vi "_RT Read XML Expt.vi"(4 "error in":errorcluster, 6 "# of Expts":i32, 7 "XML String":string) -> (0 "error out":errorcluster, 1 "Expt":T1[](array[typedef]) {"ScanType" format="%#.6g"; "Mass Range"."Res" items=["High/High", "Medium/Medium", "Low/Low", "High/Medium", "High/Low", "Medium/High", "Medium/Low", "Low/High", "Low/Medium"]}, 3 "Remaining String":string)   [LabVIEW 2015]
uses:
  Type/_XML Expt.ctl
  Type/_XML Lens.ctl
  Type/_Mass Range Property.ctl
  Type/_Mass Range Parameters.ctl
  Type/_RT Res Type.ctl
  Type/_XML Type.ctl
  _RT Global.vi
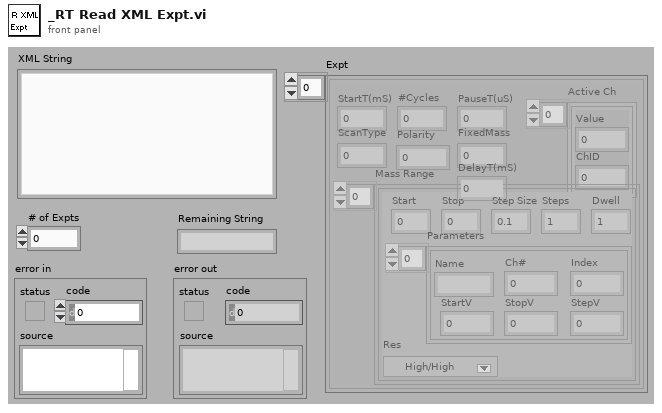
[diagram p1: front panel]
types:
  T1 = typedef "_XML Expt.ctl" = cluster{"StartT(mS)":i32, "#Cycles":i32, "PauseT(uS)":i32, "ScanType":i32, "Polarity":u8, "FixedMass":dbl, "DelayT(mS)":i32, "Active Ch":T2[], "Mass Range":T3[]}
  T2 = typedef "_XML Lens.ctl" = cluster{"Value":dbl, "ChID":u8}
  T3 = typedef "_Mass Range Property.ctl" = cluster{"Start":dbl, "Stop":dbl, "Step Size":dbl, "Steps":i32, "Dwell":dbl, "Parameters":T4[], "Res":T5}
  T4 = typedef "_Mass Range Parameters.ctl" = cluster{"Name":string, "Ch#":u8, "StartV":dbl, "StopV":dbl, "StepV":dbl, "Index":u8}
  T5 = typedef "_RT Res Type.ctl" = u16
  T6 = typedef "_XML Type.ctl" = enum16{"Configuration", "ConTable", "Method", "Experiment", "Mass Range", "Table", "LensTable", "ParamTable", "TuneParam", "MetParam", "MassRange", "LCMethod", "LCMethodFile", "RackType", "Vial", "PlatePos", "InjVol"}
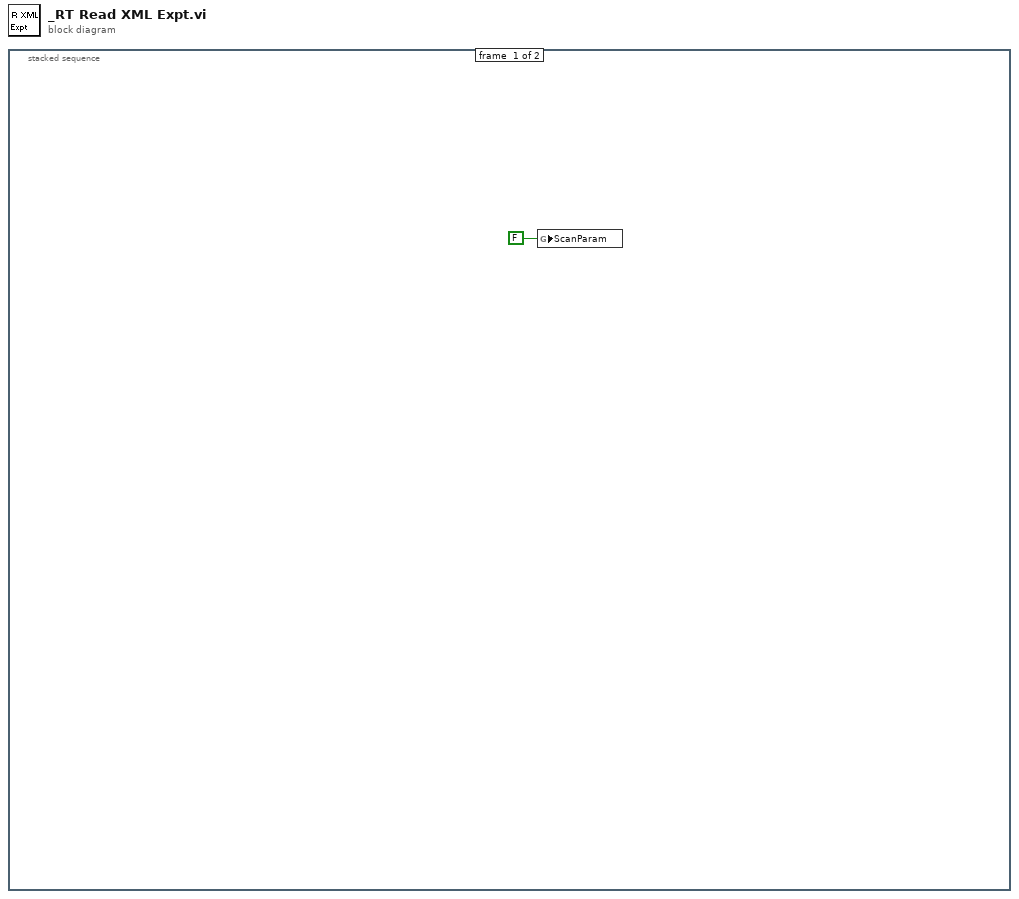
[diagram p0: block diagram]
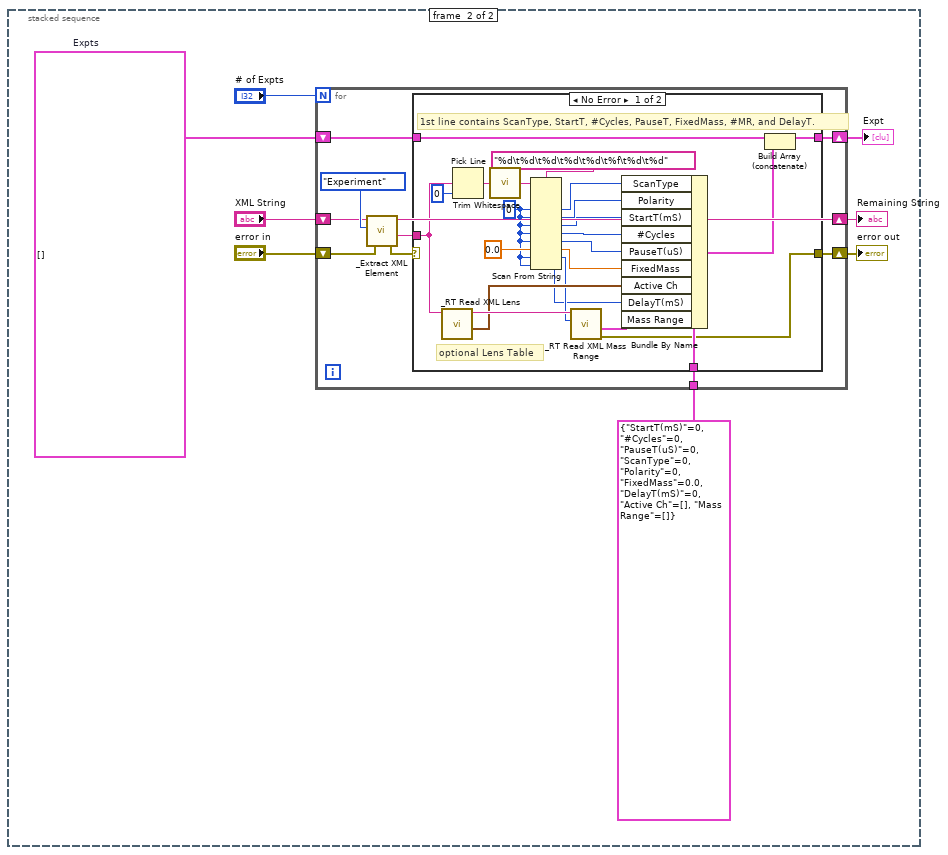
[diagram p2: hidden frame]
diagram:
  n1 = stacked-sequence {
    frame #0 {
      n2 = global write "_RT Global.vi" "ScanParam"(FALSE ("ScanParam")) -> ()
    }
    frame #1 {
      w4 = T1[] []  # Expts
      n3 = for {
        N: "# of Expts" -> [_]
        shift-right: [w13] -> w6
        shift-left: "XML String" -> [w15]
        shift-right: [w14] -> w5
        shift-left: "error in" -> [w18]
        shift-right: [w10] -> w2
        shift-left: w4 -> [w12]
        tunnel: T1 {"StartT(mS)"=0, "#Cycles"=0, "PauseT(uS)"=0, "ScanType"=0, "Polarity"=0, "FixedMass"=0.0, "DelayT(mS)"=0, "Active Ch"=[], "Mass Range"=[]} ("Expt") -> [w11]
        n4 = call "_Extract XML Element.vi"("error in"=w18, "XML Type"=_XML_Type."Experiment", "XML String"=w15) -> ("error out"=w17:errorcluster, "Element"=w16:string, "Remaining String"=w13:string)  [unwired: 2 out]
        n5 = case shown="No Error" w17 {
          selector: w17 -> [_ w44]
          tunnel: [w29 w44] -> w14
          tunnel: w16 -> [w38 _]
          tunnel: w12 -> [w33 w43]
          tunnel: w11 -> [w37 _]
          tunnel: [w31 w43] -> w10
          frame No Error {
            w22 = 0 ("Ch#")
            # "optional Lens Table"
            # "1st line contains ScanType, StartT, #Cycles, PauseT, FixedMass, #MR, and DelayT."
            n6 = call "_RT Read XML Lens.vi"("XML String"=w38) -> ("Lens"=w25:T2[], "Remaining String"=w30:string)  [unwired: 4 in, 1 out]
            n7 = Pick Line(multi-line string=w38, line index=0) -> (output string=w42:string)  [unwired: 1 out]
            n8 = call <vilib>:"Trim Whitespace.vi"("string"=w42) -> ("trimmed string"=w39:string)  [unwired: 1 in]
            n9 = Scan From String(format string="%d\t%d\t%d\t%d\t%d\t%f\t%d\t%d", input string=w39, default 1=w22, default 2=w22, default 3=w22, default 4=w22, default 5=w22, default 6=0.0 ("Ch#"), default 7=w22, default 8=w22) -> (output 1=w36:i32, output 2=w28:i32, output 3=w35:i32, output 4=w34:i32, output 5=w26:i32, output 6=w24:dbl, output 7=w23:i32, output 8=w20:i32)  [unwired: 2 in, 3 out]
            n10 = call "_RT Read XML Mass Range.vi"("# of MRs"=w23, "XML String"=w30) -> ("error out"=w29:errorcluster, "Mass Range"=w21:T3[])  [unwired: 3 in, 1 out]
            n11 = Bundle By Name(cluster=w37, "ScanType"=w36, "Polarity"=w28, "StartT(mS)"=w35, "#Cycles"=w34, "PauseT(uS)"=w26, "FixedMass"=w24, "Active Ch"=w25, "DelayT(mS)"=w20, "Mass Range"=w21) -> (w32:T1)
            n12 = Build Array (concatenate)(w33, w32) -> (w31:T1[])
          }
          frame Error {
          }
        }
      }
      "Remaining String" <- w6
      "error out" <- w5
      "Expt" <- w2
    }
  }
